vi "Main_Transmitter_dummytest.vi"(8 "error in (no error)":errorcluster, 10 "Packet Parameters in":T3={"Length of sync sequence (50)"=50, "Number of message bits"=2048, "Number of guardbits"=30, "Sync PN sequence order (31)"=31, "Number of header bits"=16, "Packet Pad [samples]"=200}, 11 "QPSK System Parameters":T4={"Samples per Symbol"=8, "symbol map"=[], "Differential PSK"=enum."enable", "PSK type"=0, "M-PSK"=8} {"PSK type" items=["normal", "shifted", "offset"]; "symbol map" format="%.3f"}) -> (0 "error out":errorcluster)   [LabVIEW 2014]
uses:
  <vilib>/addons/Modulation/Digital/General/MT Generate Bits (Galois, PN Order).vi
  <vilib>/addons/Modulation/Digital/Support/Common/Validators/mod_Generate Bits Validate.vi
  <vilib>/addons/Modulation/Analog/support/mod_Set Error Source.vi
  <vilib>/addons/Modulation/Digital/General/subVIs/mod_Generate Bits PN Sequence.vi
  <vilib>/addons/Modulation/Digital/General/MT Format Eye Diagram (complex).vi
  <instrlib>/niUSRP/niUSRP Write Tx Data (CDB Cluster).vi
  <vilib>/addons/Modulation/niDMT.lvlib
panel:
  in  "I/Q (I)":enum16{"I", "Q"}(ring) caption="Eye Diagram I/Q"
  out "Eye Diagram":cluster{"t0":dbl, "dt":dbl, "Y":dbl[]}[](graph)
  in  "autoscale":bool
  out "Constellation Graph":T1(graph)
  in  "Test Setup":T2={"Packets to send"=100, "Queue Length"=10, "PN sequence order (9)"=9}
  out "Frame transfer time [ms]":dbl
  out "Frame length [samples]":i32
  out "Effective bit rate [bits/s]":dbl
  out "Real Frames Sent":i32
  out "Blank Frames Sent":i32
  out "Time to transfer packet [ms]":dbl
  in  "stop 2":bool caption="stop"
  in  "Bits per sample":i32=16
  in  "Audio record time/delay (ms)":i32=200
  in  "Audio sample rate (Fs)":i32=6000
  in  "filter parameters":T5={"Alpha"=0.5, "Filter Length"=6, "TX Filter"=enum."Root Raised Cos"} {"Alpha" format="%.2f"}
  in  "USRP IP address":refnum<k15>="192.168.10.1"
  in  "Tx Parameters":T6={"Tx IQ Sampling\nRate [s/sec]"=400000.0, "Tx Frequency [Hz]"=2450000000.0, "Tx Gain [dB]"=0.0, "Tx Antenna"="TX1"} {"Tx Gain [dB]" format="%#.6p"; "Tx Frequency [Hz]" format="%#.6p"; "Tx IQ Sampling\nRate [s/sec]" format="%#.6p"}
  out "Actual Tx Parameters":T6={"Tx IQ Sampling\nRate [s/sec]"=400000.0, "Tx Frequency [Hz]"=915000000.0, "Tx Gain [dB]"=0.0, "Tx Antenna"="TX1"} {"Tx Gain [dB]" format="%#.6p"; "Tx Frequency [Hz]" format="%#.6p"; "Tx IQ Sampling\nRate [s/sec]" format="%#.6p"}
  # "Calculated values"
  # "Measurements"
  # "Graph Setup"
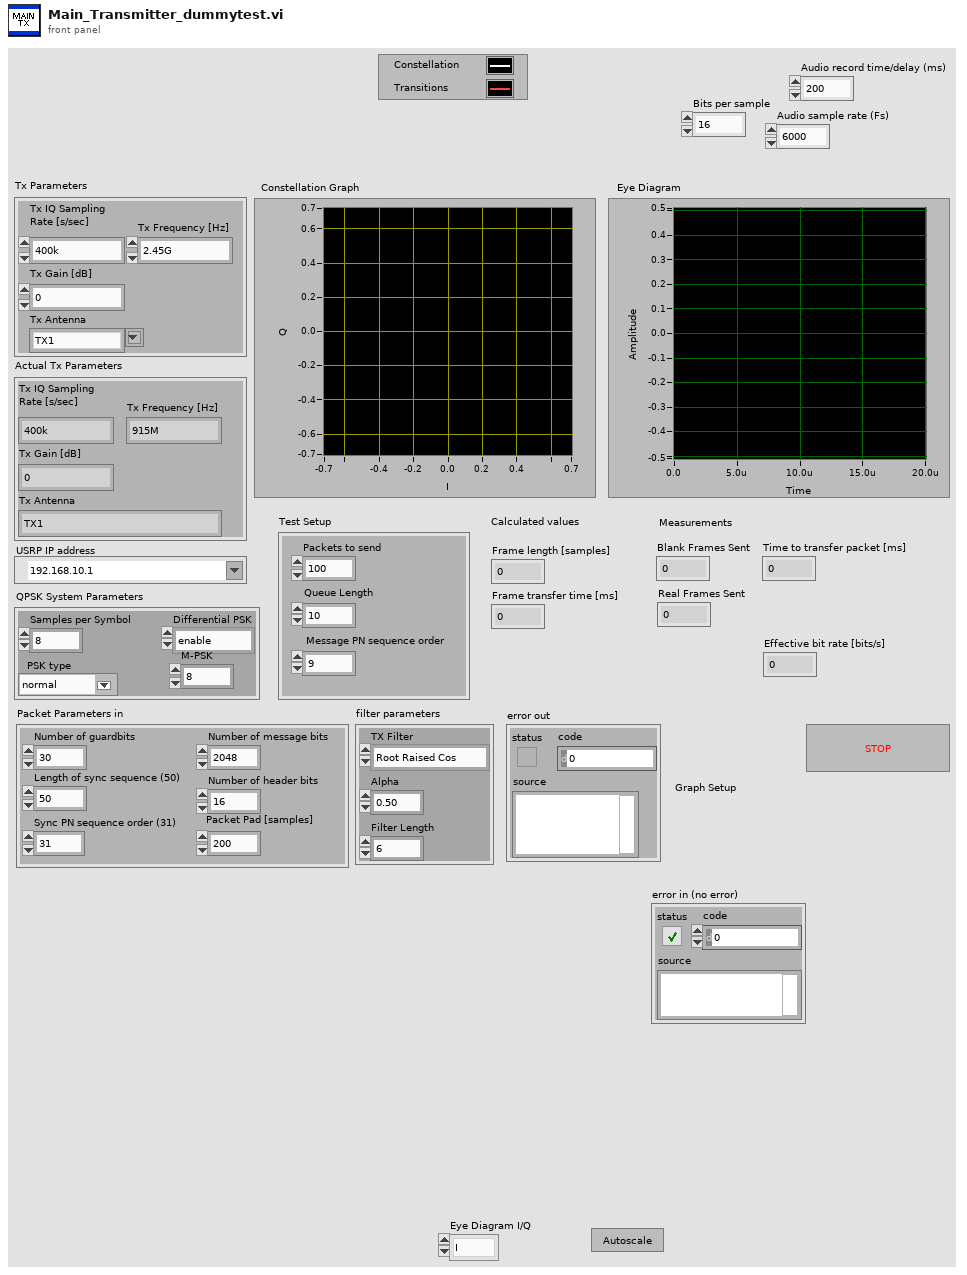
[diagram p1: front panel]
types:
  T1 = cluster{"Decimated Array":dbl[], "Decimated Array":dbl[]}[]
  T2 = cluster{"Packets to send":i32, "Queue Length":i32, "PN sequence order (9)":i32}
  T3 = cluster{"Length of sync sequence (50)":i32, "Number of message bits":i32, "Number of guardbits":i32, "Sync PN sequence order (31)":i32, "Number of header bits":i32, "Packet Pad [samples]":i32}
  T4 = cluster{"Samples per Symbol":i32, "symbol map":cdb[], "Differential PSK":enum16{"disable", "enable"}, "PSK type":u16, "M-PSK":i32}
  T5 = cluster{"Alpha":dbl, "Filter Length":i32, "TX Filter":enum16{"none", "Raised Cosine", "Root Raised Cos", "Gaussian"}}
  T6 = cluster{"Tx IQ Sampling\nRate [s/sec]":dbl, "Tx Frequency [Hz]":dbl, "Tx Gain [dB]":dbl, "Tx Antenna":string}
  T7 = cluster{"samples per symbol (16)":i32, "symbol map":cdb[], "differential PSK":enum16{"disable", "enable"}, "PSK type":u16}
  T8 = cluster{"s? t:f":cluster{"t0":dbl, "dt":dbl, "Y":cdb[]}, i32}
  T9 = typedef "niAMT.lvlib/Complex Data Waveform.ctl" = cluster{"t0":dbl, "dt":dbl, "Y":cdb[]}
  T10 = cluster{"constellation":dbl[], "oversampled data":dbl[]}[]
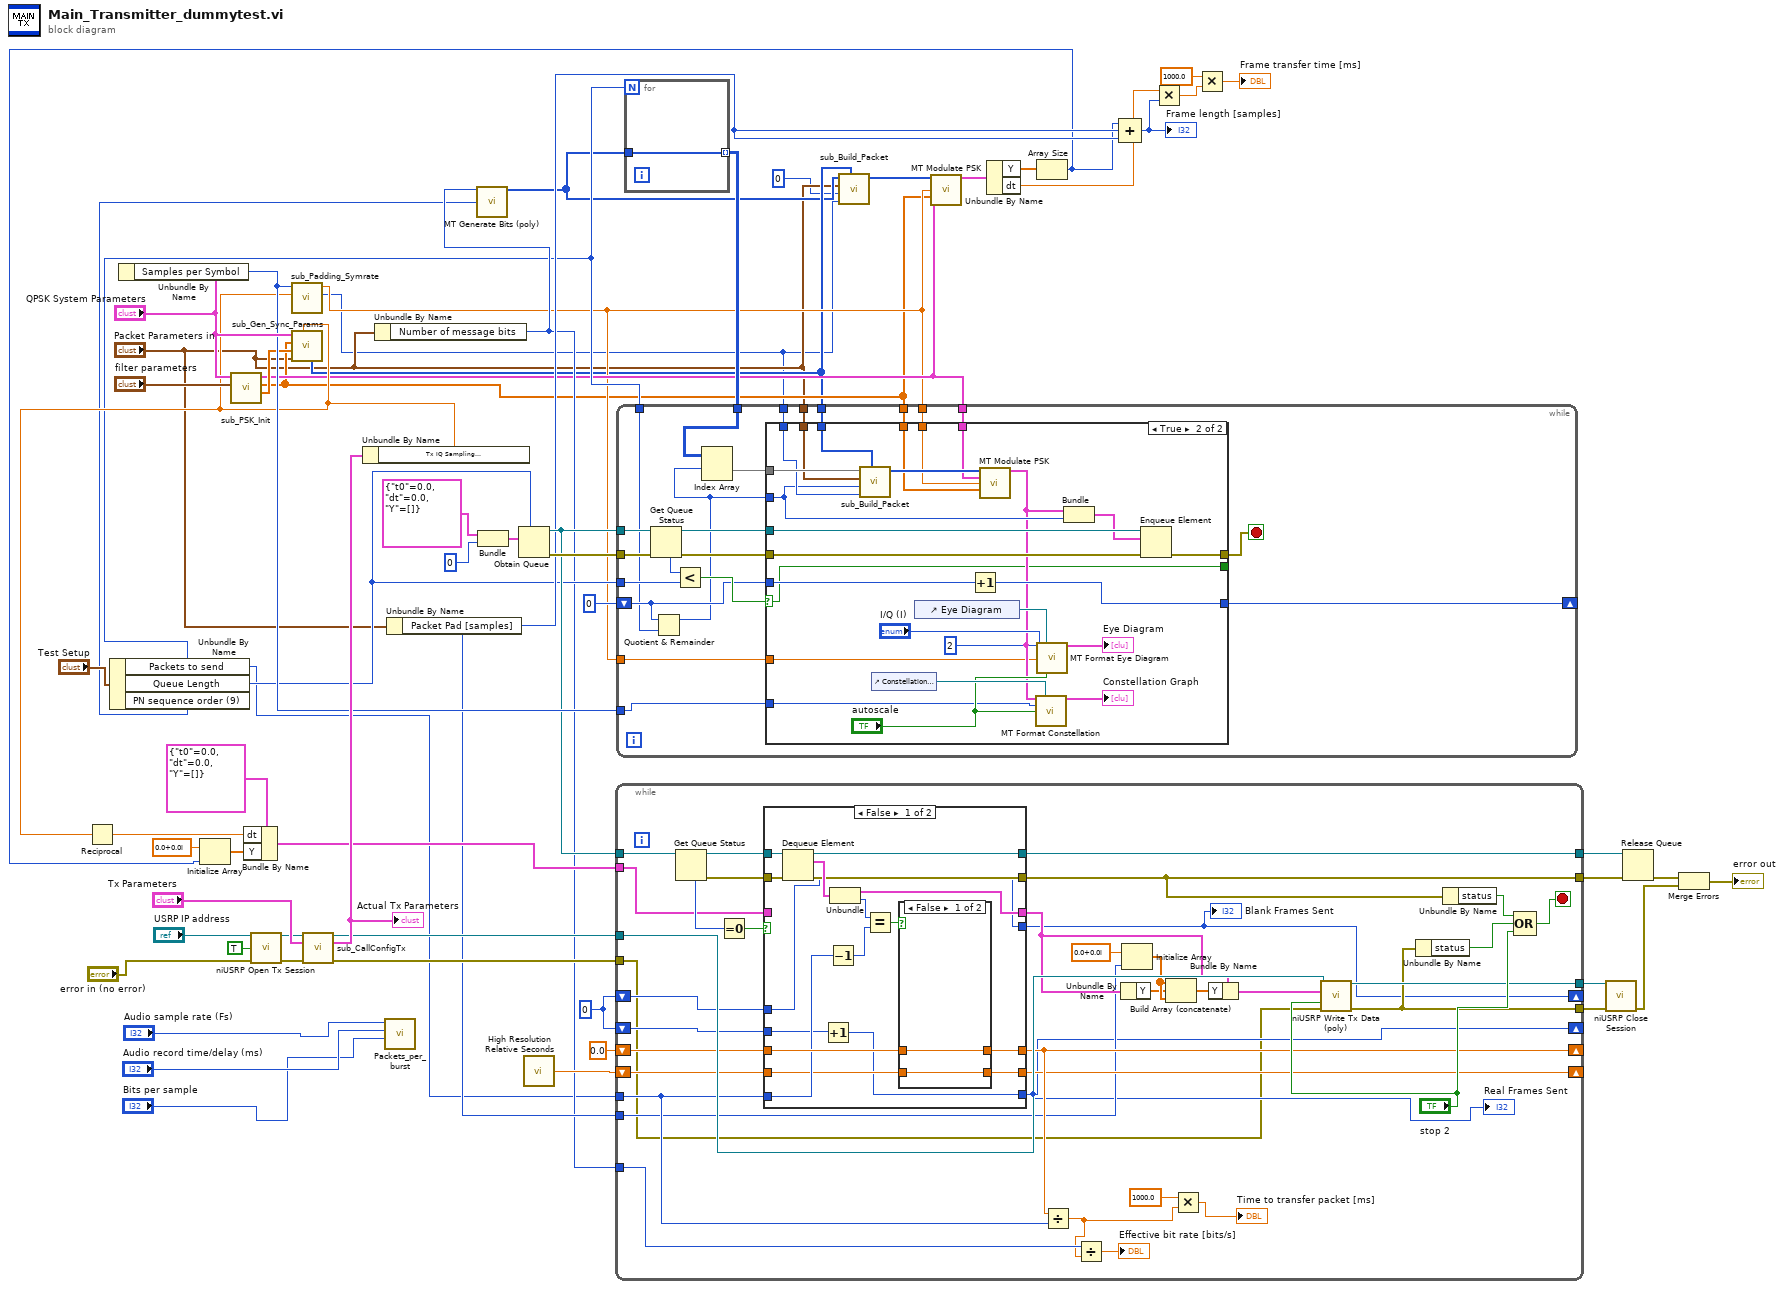
[diagram p0: block diagram]
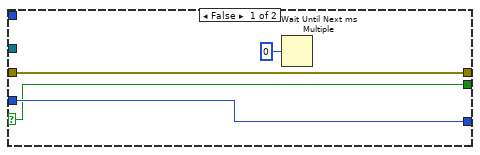
[diagram p2: hidden frame]
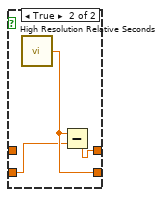
[diagram p3: hidden frame]
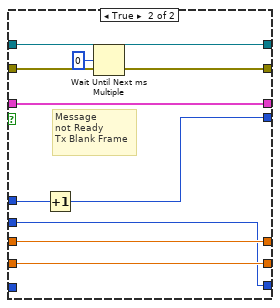
[diagram p4: hidden frame]
diagram:
  w27 = 0
  n1 = Unbundle By Name("Test Setup") -> ("Packets to send"=w15:i32, "Queue Length"=w21:i32, "PN sequence order (9)"=w16:i32)
  n2 = Unbundle By Name("QPSK System Parameters") -> ("Samples per Symbol"=w43:i32)
  n3 = call "sub_PSK_Init.vi"("filter parameters in"="filter parameters", "QPSK System Parameters in"="QPSK System Parameters") -> ("matched filter coefficients"=w19:dbl[], "pulse shaping filter coefficients"=w10:dbl[], "PSK system parameters"=w12:T7)  [unwired: 7 in]
  n4 = call <instrlib>:"niUSRP Open Tx Session.vi"("device names"="USRP IP address", "reset"=TRUE, "error in (no error)"="error in (no error)") -> ("session handle out"=w61:refnum<k15>, "error out"=w60:errorcluster)  [unwired: 11 in]
  n5 = call "sub_CallConfigTx.vi"("session handle"=w61, "Tx Parameters"="Tx Parameters", "error in"=w60) -> ("session handle out"=w55:refnum<k15>, "Actual Tx Parameters"=w56:T6, "error out"=w57:errorcluster)  [unwired: 10 in]
  "Actual Tx Parameters" <- w56
  n6 = Unbundle By Name(w56) -> ("Tx IQ Sampling\nRate [s/sec]"=w18:dbl)
  n7 = Reciprocal(x=w18) -> (1/x=w39:dbl)
  n8 = call "sub_Padding_Symrate.vi"("Tx IQ Sampling\nRate [s/sec]"=w18, "Samples per Symbol"=w43) -> ("Padding Bits"=w5:i32, "Symbol Rate"=w11:dbl)  [unwired: 8 in]
  n9 = call "sub_Gen_Sync_Params.vi"("IQ Sampling\nRate [s/sec]"=w18, "Packet Parameters in"="Packet Parameters in", "matched filter coefficients"=w19, "pulse shaping filter coefficients"=w10, "QPSK System Parameters in"="QPSK System Parameters") -> ("Sync Sequence Bitstream"=w9:i8[])  [unwired: 2 in, 4 out]
  n10 = Unbundle By Name("Packet Parameters in") -> ("Number of message bits"=w17:i32)
  n11 = call "Packets_per_burst.vi"("Bits per sample"="Bits per sample", "Audio record time/delay (ms)"="Audio record time/delay (ms)", "Audio sample rate (Fs)"="Audio sample rate (Fs)") -> ()  [unwired: 8 in, 1 out]
  n12 = Unbundle By Name("Packet Parameters in") -> ("Packet Pad [samples]"=w23:i32)
  n13 = call-poly <vilib>:"MT Generate Bits (poly).vi"("total bits (128)"=w17, "PN sequence order (9)"=w16) -> ("output bit stream"=w8:i8[])  [unwired: 11 in, 2 out]
  n14 = Bundle("s? t:f"=cluster{"t0":dbl, "dt":dbl, "Y":cdb[]} {"t0"=0.0, "dt"=0.0, "Y"=[]}, 0) -> (w47:T8)  [unwired: 1 in]
  n15 = Obtain Queue(max queue size (-1, unlimited)=w21, element data type=w47) -> (queue out=w42:refnum<queue>, error out=w45:errorcluster)  [unwired: 3 in, 1 out]
  n16 = call <vilib>:"High Resolution Relative Seconds.vi"() -> ("relative seconds"=w29:dbl)
  n17 = for {
    N: w15 -> [_]
    tunnel: w8 -> [w63]
    tunnel: [w63] -> w14 mode=indexing
  }
  n18 = while {
    tunnel: w42 -> [w81]
    tunnel: w45 -> [w80]
    tunnel: w21 -> [w79]
    tunnel: w43 -> [w64]
    tunnel: w15 -> [w76]
    shift-right: [w75] -> _
    shift-left: 0 -> [w78]
    tunnel: w11 -> [w65]
    tunnel: w14 -> [w74]
    tunnel: w9 -> [w72]
    tunnel: "Packet Parameters in" -> [w71]
    tunnel: w5 -> [w69]
    tunnel: w12 -> [w68]
    tunnel: w11 -> [w67]
    tunnel: w10 -> [w66]
    stop <- w77 stop-if-true
    n19 = Get Queue Status(queue=w81, error in (no error)=w80) -> (queue out=w85:refnum<queue>, error out=w82:errorcluster, # elements in queue=w84:i32)  [unwired: 1 in, 5 out]
    n20 = Quotient & Remainder(x=w78, y=w76) -> (x-y*floor(x/y)=w70:i32)  [unwired: 1 out]
    n21 = Less?(x=w84, y=w79) -> (x < y?=w83:bool)
    n22 = Index Array(array=w74, index (row)=w70) -> (element=w73:i8[])  [unwired: 1 in]
    n23 = case shown="True" w83 {
      selector: w83 -> [w86 w90]
      tunnel: w82 -> [w87 w115]
      tunnel: w85 -> [_ w114]
      tunnel: [w87 w113] -> w77
      tunnel: w78 -> [w89 w112]
      tunnel: [w89 w111] -> w75
      tunnel: w73 -> [_ w110]
      tunnel: w72 -> [_ w109]
      tunnel: w71 -> [_ w108]
      tunnel: w70 -> [_ w102]
      tunnel: w69 -> [_ w107]
      tunnel: w68 -> [_ w105]
      tunnel: w67 -> [_ w104]
      tunnel: w66 -> [_ w103]
      tunnel: w65 -> [_ w92]
      tunnel: w64 -> [_ w91]
      tunnel: [w86 w90] -> _
      frame False {
        n24 = Wait Until Next ms Multiple(millisecond multiple=u32 0) -> ()  [unwired: 1 out]
      }
      frame True {
        n25 = call "sub_Build_Packet.vi"("Sync Sequence Bitstream"=w109, "Cyclic Padding Bits"=w107, "Packet number"=w102, "Packet Parameters in"=w108, "Input Message"=w110) -> ("Packet out"=w106:i8[])  [unwired: 6 in]
        n26 = control-ref of="Constellation Graph"() -> (w97:refnum<vi>)
        n27 = control-ref of="Eye Diagram"() -> (w99:refnum<vi>)
        n28 = Increment(x=w112) -> (x+1=w111:i32)
        n29 = call <vilib>:"MT Modulate PSK.vi"("input bit stream"=w106, "PSK system parameters"=w105, "symbol rate (Hz)"=w104, "pulse shaping filter coefficients"=w103) -> ("output complex waveform"=w93:T9)  [unwired: 9 in, 2 out]
        n30 = call <vilib>:"MT Format Constellation.vi"("waveform"=w93, "constellation reference"=w97, "samples per symbol"=w91, "autoscale"="autoscale") -> ("constellation graph"=→"Constellation Graph":T10)  [unwired: 1 in, 10 out]
        n31 = call-poly <vilib>:"MT Format Eye Diagram.vi"("waveform"=w93, "eye diagram reference"=w99, "symbol rate (Hz)"=w92, "eye length"=2, "I/Q (I)"="I/Q (I)", "autoscale"="autoscale") -> ("eye diagram"=→"Eye Diagram":cluster{"t0":dbl, "dt":dbl, "Y":dbl[]}[])  [unwired: 1 in, 8 out]
        n32 = Bundle("output complex waveform"=w93, w102) -> (w101:cluster{"output complex waveform":T9, i32})  [unwired: 1 in]
        n33 = Enqueue Element(queue=w114, element=w101, error in (no error)=w115) -> (error out=w113:errorcluster)  [unwired: 1 in, 2 out]
      }
    }
  }
  n34 = call "sub_Build_Packet.vi"("Sync Sequence Bitstream"=w9, "Cyclic Padding Bits"=w5, "Packet number"=i16 0, "Packet Parameters in"="Packet Parameters in", "Input Message"=w8) -> ("Packet out"=w13:i8[])  [unwired: 6 in]
  n35 = call <vilib>:"MT Modulate PSK.vi"("input bit stream"=w13, "PSK system parameters"=w12, "symbol rate (Hz)"=w11, "pulse shaping filter coefficients"=w10) -> ("output complex waveform"=w3:T9)  [unwired: 9 in, 2 out]
  n36 = Unbundle By Name(w3) -> ("Y"=w4:cdb[], "dt"=w1:dbl)
  n37 = Array Size(array=w4) -> (size(s)=w2:i32)
  n38 = Initialize Array(cdb 0.0+0.0i ("element"), w2) -> (w40:cdb[])
  n39 = Bundle By Name(cluster=cluster{"t0":dbl, "dt":dbl, "Y":cdb[]} {"t0"=0.0, "dt"=0.0, "Y"=[]} ("s? t:f"), "dt"=w39, "Y"=w40) -> (w37:cluster{"t0":dbl, "dt":dbl, "Y":cdb[]})
  n40 = while {
    tunnel: w57 -> [w116]
    tunnel: w55 -> [w143]
    tunnel: w42 -> [w145]
    tunnel: w37 -> [w144]
    tunnel: [w141] -> w33
    tunnel: [w140] -> w32
    tunnel: [w139] -> w31
    tunnel: [w138] -> w30
    shift-right: [w136] -> _
    shift-left: 0.0 -> [w137]
    tunnel: w15 -> [w135]
    shift-right: [w134] -> _
    shift-left: w29 -> [w133]
    shift-right: [w120] -> _
    shift-left: w27 -> [w132]
    shift-right: [w119] -> _
    shift-left: w27 -> [w131]
    tunnel: w17 -> [w130]
    tunnel: w23 -> [w124]
    stop <- w142 stop-if-true
    n41 = Get Queue Status(queue=w145) -> (queue out=w150:refnum<queue>, error out=w149:errorcluster, # elements in queue=w152:i32)  [unwired: 2 in, 5 out]
    n42 = Equal To 0?(x=w152) -> (x = 0?=w151:bool)
    n43 = case shown="False" w151 {
      tunnel: w144 -> [_ w183]
      tunnel: [w165 w183] -> w125
      tunnel: [w169 w181] -> w141
      tunnel: [w164 w182] -> w140
      tunnel: w150 -> [w168 w181]
      tunnel: w149 -> [w167 w182]
      tunnel: w137 -> [w161 w179]
      tunnel: [w160 w179] -> w136
      tunnel: w135 -> [w158 _]
      tunnel: [w157 w178] -> w134
      tunnel: w133 -> [w156 w178]
      tunnel: w132 -> [w155 w177]
      tunnel: [w155 w176] -> w120
      tunnel: w131 -> [w154 w175]
      tunnel: [w153 w175] -> w119
      frame False {
        n44 = Dequeue Element(queue=w168, error in (no error)=w167) -> (queue out=w169:refnum<queue>, element=w166:T8, error out=w164:errorcluster)  [unwired: 1 in, 1 out]
        n45 = Increment(x=w154) -> (x+1=w153:i32)
        n46 = Decrement(x=w158) -> (x-1=w159:i32)
        n47 = Unbundle(w166) -> ("s? t:f"=w165:cluster{"t0":dbl, "dt":dbl, "Y":cdb[]}, w162:i32)
        n48 = Equal?(x=w162, y=w159) -> (x = y?=w163:bool)
        n49 = case shown="False" w163 {
          tunnel: w161 -> [w170 _]
          tunnel: [w170 w174] -> w160
          tunnel: [w171 w173] -> w157
          tunnel: w156 -> [w171 w172]
          frame False {
          }
          frame True {
            n50 = call <vilib>:"High Resolution Relative Seconds.vi"() -> ("relative seconds"=w173:dbl)
            n51 = Subtract(x=w173, y=w172) -> (x-y=w174:dbl)
          }
        }
      }
      frame True {
        # "Message\nnot Ready\nTx Blank Frame"
        n52 = Increment(x=w177) -> (x+1=w176:i32)
        n53 = Wait Until Next ms Multiple(millisecond multiple=u32 0) -> ()  [unwired: 1 out]
      }
    }
    "Blank Frames Sent" <- w120
    "Real Frames Sent" <- w119
    n54 = Divide(x=w136, y=w135) -> (x/y=w122:dbl)
    n55 = Divide(x=w130, y=w122) -> (x/y=→"Effective bit rate [bits/s]":dbl)
    n56 = Unbundle By Name(w125) -> ("Y"=w126:cdb[])
    n57 = Initialize Array(cdb 0.0+0.0i ("element"), w124) -> (w127:cdb[])
    n58 = Build Array (concatenate)(w127, w126, w127) -> (w129:cdb[])
    n59 = Multiply(x=1000.0, y=w122) -> (x*y=→"Time to transfer packet [ms]":dbl)
    n60 = Bundle By Name(cluster=w125, "Y"=w129) -> (w121:cluster{"t0":dbl, "dt":dbl, "Y":cdb[]})
    n61 = call-poly <instrlib>:"niUSRP Write Tx Data (poly).vi"("session handle"=w143, "data"=w121, "end of data?"="stop 2", "error in (no error)"=w116) -> ("session handle out"=w139:refnum<k15>, "error out"=w138:errorcluster)  [unwired: 10 in]
    n62 = Unbundle By Name(w138) -> ("status"=w148:bool)
    n63 = Unbundle By Name(w140) -> ("status"=w146:bool)
    n64 = Compound Arithmetic op=OR(w146, w148, "stop 2") -> (w142:bool)
  }
  n65 = Compound Arithmetic op=ADD(w2, w23, w23) -> (w20:i32)
  "Frame length [samples]" <- w20
  n66 = Multiply(x=w1, y=w20) -> (x*y=w26:dbl)
  n67 = Multiply(x=1000.0, y=w26) -> (x*y=→"Frame transfer time [ms]":dbl)
  n68 = call <instrlib>:"niUSRP Close Session.vi"("session handle"=w31, "error in (no error)"=w30) -> ("error out"=w35:errorcluster)  [unwired: 13 in]
  n69 = Release Queue(queue=w33, error in (no error)=w32) -> (error out=w36:errorcluster)  [unwired: 3 out]
  n70 = Merge Errors(w36, w35) -> (→"error out":errorcluster)
